vi "XyBarGraphTests.vi"() -> ()   [LabVIEW 2014]
panel:
  in  "stop":bool
  out "XY Graph":cluster{i32[], "Y-axis":dbl[]}(graph)
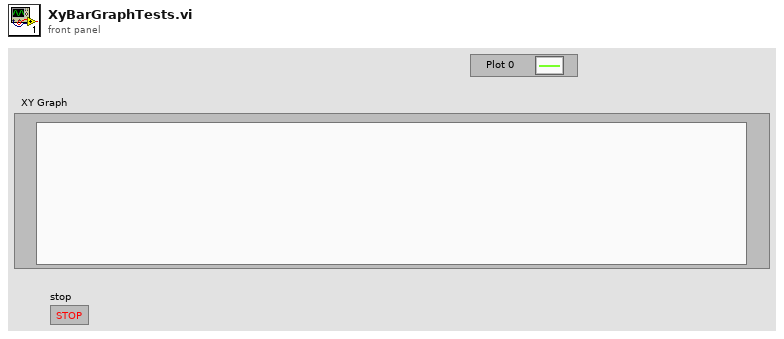
[diagram p1: front panel]
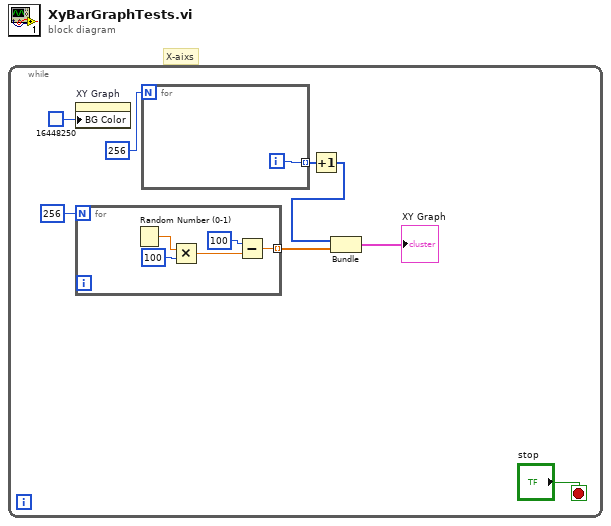
[diagram p0: block diagram]
diagram:
  # "X-aixs"
  n1 = while {
    stop <- "stop" stop-if-true
    n2 = property on="XY Graph" class="XYGraph (strict)"("BG Color"=u32 16448250) -> ()  [unwired: 2 in, 2 out]
    n3 = for {
      N: 256 -> [_]
      tunnel: [w9] -> w6 mode=indexing
      n4 = Random Number (0-1)() -> (number: 0 to 1=w13:dbl)
      n5 = Multiply(x=w13, y=100) -> (x*y=w10:dbl)
      n6 = Subtract(x=100, y=w10) -> (x-y=w9:dbl)
    }
    n7 = for {
      N: 256 -> [_]
      tunnel: [w14] -> w3 mode=indexing
      i -> [w14]
    }
    n8 = Increment(x=w3) -> (x+1=w2:i32[])
    n9 = Bundle(w2, w6) -> (→"XY Graph":cluster{i32[], dbl[]})  [unwired: 1 in]
  }
